vi "Queues FGV.vi"(7 "Action":T1, 8 "Error In":errorcluster) -> (0 "Error Out":errorcluster)   [LabVIEW 2019, in "Queues.lvlib"]
uses:
  Queues.lvlib
  Queues FGV Action.ctl
  Message Cluster.ctl
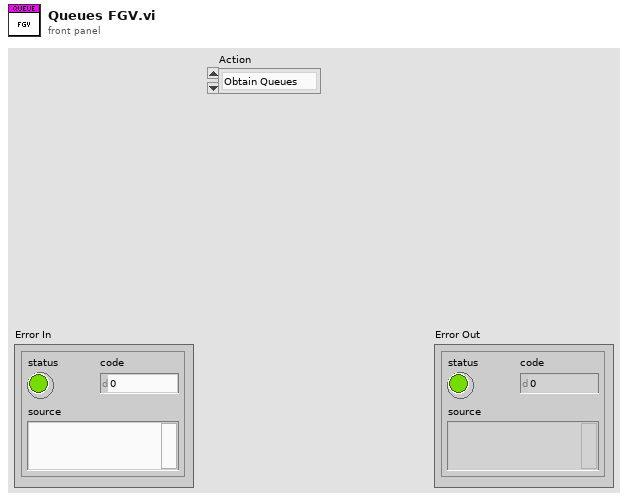
[diagram p1: front panel]
types:
  T1 = typedef "Queues.lvlib/Queues FGV Action.ctl" = enum16{"Obtain Queues", "Release Queues"}
  T2 = typedef "Queues.lvlib/Message Cluster.ctl" = cluster{"State":string, "Data":variant}
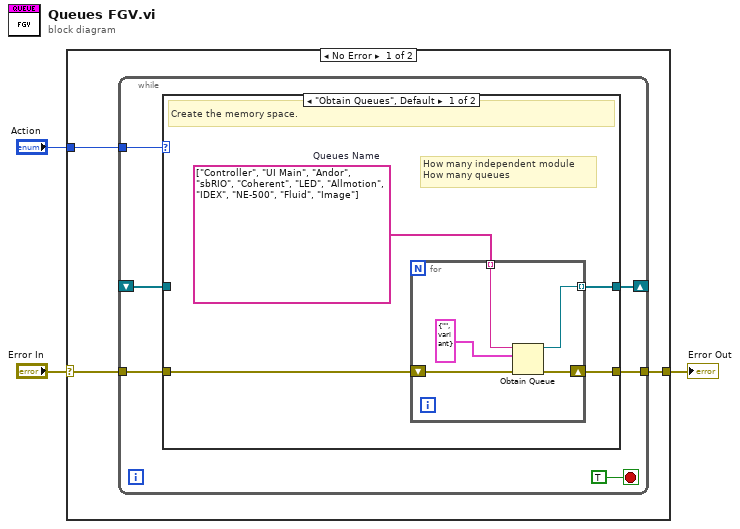
[diagram p0: block diagram]
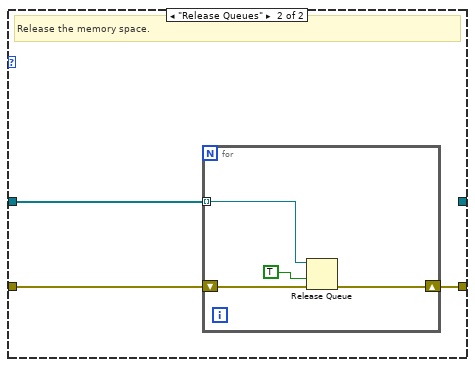
[diagram p2: hidden frame]
diagram:
  n1 = case shown="No Error" "Error In" {
    selector: "Error In" -> [w5 w29]
    tunnel: "Action" -> [w6 _]
    tunnel: [w4 w29] -> w1
    frame No Error {
      n2 = while {
        tunnel: w6 -> [w12]
        shift-right: [w11] -> _
        shift-left: _ -> [w10]
        tunnel: w5 -> [w9]
        tunnel: [w8] -> w4
        stop <- TRUE stop-if-true
        n3 = case shown="\"Obtain Queues\", Default" w12 {
          tunnel: [w14 _] -> w11
          tunnel: w10 -> [_ w22]
          tunnel: w9 -> [w16 w24]
          tunnel: [w15 w23] -> w8
          frame "Obtain Queues", Default {
            w13 = string[] ["Controller", "UI Main", "Andor", "sbRIO", "Coherent", "LED", "Allmotion", "IDEX", "NE-500", "Fluid", "Image"]  # Queues Name
            # "How many independent module\nHow many queues"
            # "Create the memory space."
            n4 = for {
              shift-right: [w20] -> w15
              shift-left: w16 -> [w21]
              tunnel: [w19] -> w14 mode=indexing
              tunnel: w13 -> [w17] mode=indexing
              n5 = Obtain Queue(name (unnamed)=w17, element data type=T2 {"State"="", "Data"=variant} ("Message"), error in (no error)=w21) -> (queue out=w19:refnum<queue>, error out=w20:errorcluster)  [unwired: 2 in, 1 out]
            }
          }
          frame "Release Queues" {
            # "Release the memory space."
            n6 = for {
              shift-right: [w27] -> w23
              shift-left: w24 -> [w28]
              tunnel: w22 -> [w26] mode=indexing
              n7 = Release Queue(queue=w26, force destroy? (F)=TRUE, error in (no error)=w28) -> (error out=w27:errorcluster)  [unwired: 2 out]
            }
          }
        }
      }
    }
    frame Error {
    }
  }
  "Error Out" <- w1
